vi "Handle Error.vi"(8 "error in (no error)":errorcluster, 11 "Ancestor in":refnum<class "Ancestor.lvclass">) -> (0 "error out":errorcluster, 2 "stop actor?":bool=TRUE, 3 "Ancestor out":refnum<class "Ancestor.lvclass">)   [LabVIEW 2026, in "TALOS.lvlib" / "Ancestor.lvlib" / "Ancestor.lvclass"]
doc: "(<B>Filename</B>: Actor Framework.lvlib:Actor.lvclass:Handle Error.vi)\n\nDefines how the actor handles an error that occurred while processing a message. By default, this method does nothing except stop the actor."
uses:
  Ancestor.lvclass
  C:/LabVIEW Code/TALOS/builds/Actor Framework PPL/Actor Framework.lvlibp/1abvi3w/vi.lib/ActorFramework/Actor/Actor.lvclass
  Guardian/Guardian/Guardian.lvclass
  C:/LabVIEW Code/TALOS/talos/Ancestor/Ancestor/Ancestor.lvclass
  builds/Actor Framework PPL/Actor Framework.lvlibp/1abvi3w/vi.lib/ActorFramework/Message Enqueuer/Message Priority.ctl
  builds/Actor Framework PPL/Actor Framework.lvlibp/1abvi3w/vi.lib/ActorFramework/Message Enqueuer/Enqueue.vi
  Guardian/Guardian Messages/Raise Abort Msg/Raise Abort Msg.lvclass
  builds/Actor Framework PPL/Actor Framework.lvlibp/1abvi3w/vi.lib/ActorFramework/Actor/Actor.lvclass
  builds/Actor Framework PPL/Actor Framework.lvlibp/1abvi3w/vi.lib/ActorFramework/Message Enqueuer/Message Enqueuer.lvclass
  <vilib>/MultiError/TokenizeJSON/Multi Error Cluster.lvlib
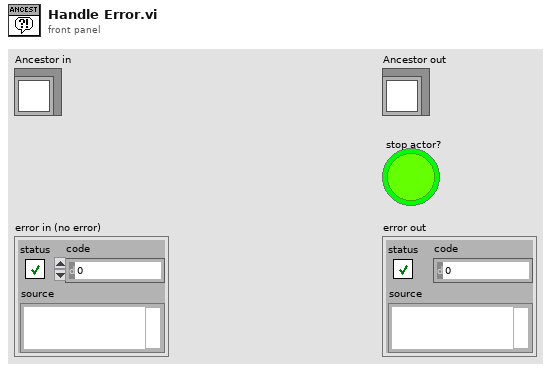
[diagram p1: front panel]
types:
  T1 = typedef "Actor Framework.lvlibp/Message Enqueuer.lvclass/Message Priority.ctl" = enum16{"Low", "Normal", "High"}
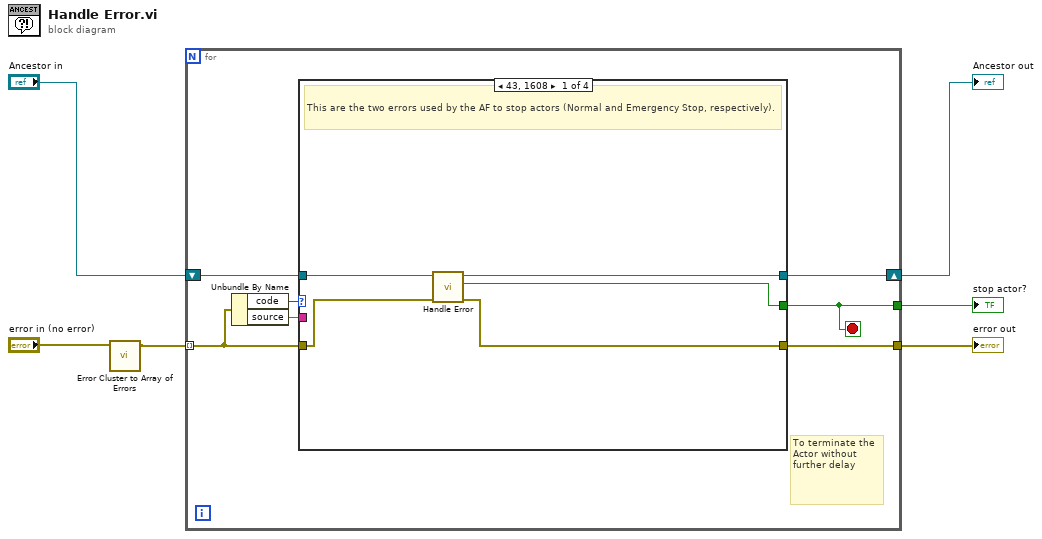
[diagram p0: block diagram]
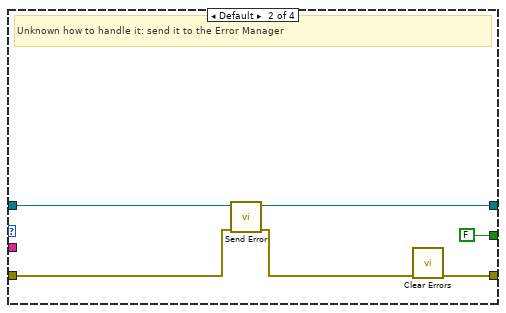
[diagram p2: hidden frame]
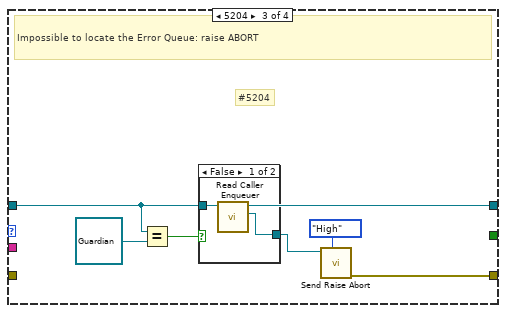
[diagram p3: hidden frame]
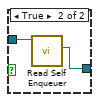
[diagram p4: hidden frame]
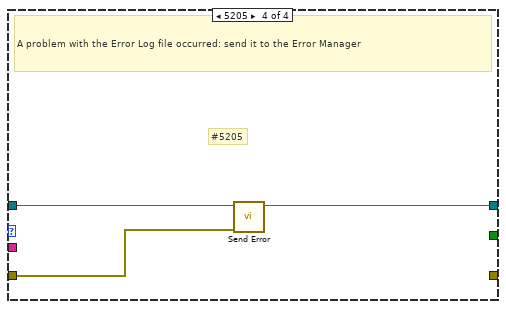
[diagram p5: hidden frame]
diagram:
  n1 = call <vilib>:"Error Cluster to Array of Errors.vi"("error"="error in (no error)") -> ("array of errors"=w1:errorcluster[])  [unwired: 10 in]
  n2 = for {
    tunnel: [w7] -> w4
    tunnel: [w11] -> w3
    tunnel: w1 -> [w8] mode=indexing
    shift-right: [w12] -> w5
    shift-left: "Ancestor in" -> [w13]
    stop <- w7 stop-if-true
    # "To terminate the Actor without further delay"
    n3 = Unbundle By Name(w8) -> ("code"=w10:i32, "source"=w9:string)
    n4 = case shown="43, 1608" w10 {
      tunnel: w8 -> [w18 w21 _ w36]
      tunnel: [w14 w19 w25 _] -> w11
      tunnel: w13 -> [w17 w22 w28 w37]
      tunnel: [w16 FALSE ("stop actor?") _ _] -> w7
      tunnel: [w15 w23 w28 w35] -> w12
      tunnel: w9 -> [_ _ _ _]
      frame 43, 1608 {
        # "This are the two errors used by the AF to stop actors (Normal and Emergency Stop, respectively)."
        n5 = call-parent "Handle Error.vi"("error in (no error)"=w18, "Actor in"=w17) -> ("error out"=w14:errorcluster, "stop actor?"=w16:bool, "Actor out"=w15:refnum<class "Ancestor.lvclass">)  [unwired: 7 in]
      }
      frame Default {
        # "Unknown how to handle it: send it to the Error Manager"
        n6 = call-dynamic "Send Error.vi"("error in (no error)"=w21, "Ancestor in"=w22) -> ("error out"=w20:errorcluster, "Ancestor out"=w23:refnum<class "Ancestor.lvclass">)  [unwired: 8 in]
        n7 = call <vilib>:"Clear Errors.vi"("error in (no error)"=w20) -> ("error out"=w19:errorcluster)  [unwired: 5 in, 1 out]
      }
      frame 5204 {
        # "#5204"
        # "Impossible to locate the Error Queue: raise ABORT"
        n8 = Equal?(x=w28, y=refnum<class "Guardian.lvclass"> refnum ("TALOS.lvlib:Guardian.lvlib:Guardian.lvclass")) -> (x = y?=w29:bool)
        n9 = case shown="False" w29 {
          tunnel: w28 -> [w32 w34]
          tunnel: [w31 w33] -> w27
          frame False {
            n10 = call "Read Caller Enqueuer.vi"("Actor"=w32) -> ("Caller Enqueuer"=w31:refnum<class "Message Enqueuer.lvclass">)  [unwired: 10 in]
          }
          frame True {
            n11 = call "Read Self Enqueuer.vi"("Actor"=w34) -> ("Self Enqueuer"=w33:refnum<class "Message Enqueuer.lvclass">)  [unwired: 10 in]
          }
        }
        n12 = call "Send Raise Abort.vi"("Message Priority (Normal)"=Message_Priority."High", "Message Enqueuer"=w27) -> ("error out"=w25:errorcluster)  [unwired: 8 in, 1 out]
      }
      frame 5205 {
        # "#5205"
        # "A problem with the Error Log file occurred: send it to the Error Manager"
        n13 = call-dynamic "Send Error.vi"("error in (no error)"=w36, "Ancestor in"=w37) -> ("Ancestor out"=w35:refnum<class "Ancestor.lvclass">)  [unwired: 8 in, 1 out]
      }
    }
  }
  "Ancestor out" <- w5
  "error out" <- w3
  "stop actor?" <- w4
